vi "serial.Read.vi"(8 "error in":errorcluster, 11 "VISA in":refnum<visa-resource-name>) -> (0 "error out":errorcluster, 2 "msg":string)   [LabVIEW 2020]
uses:
  ecc83fa6-065f-4ed5-ad9c-77edae2b4f3b.vi
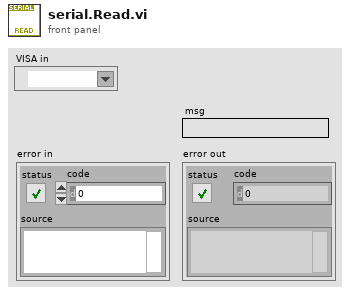
[diagram p1: front panel]
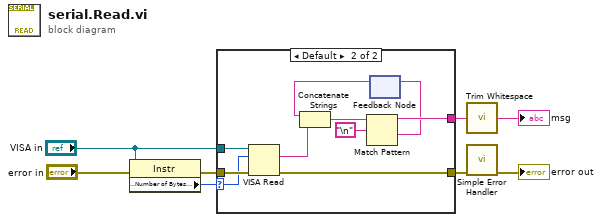
[diagram p0: block diagram]
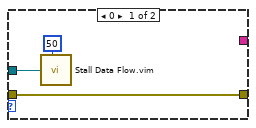
[diagram p2: hidden frame]
diagram:
  n1 = property class="Instr"(reference="VISA in", error in="error in") -> (error out=w6:errorcluster, "Serial Settings:Number of Bytes at Serial Port"=w7:u32)  [unwired: 1 out]
  n2 = case shown="Default" w7 {
    selector: w7 -> [_ w19]
    tunnel: w6 -> [w9 w21]
    tunnel: "VISA in" -> [w11 w20]
    tunnel: [w9 w18] -> w4
    tunnel: [_ w16] -> w3
    frame 0 {
      n3 = call "Stall Data Flow.vim"("value in"=w11, "milliseconds to wait"=u32 50) -> ()  [unwired: 2 out]
    }
    frame Default {
      n4 = VISA Read(VISA resource name=w20, byte count=w19, error in (no error)=w21) -> (read buffer=w13:string, error out=w18:errorcluster)  [unwired: 2 out]
      n5 = feedback #1() -> (w12:string)  [unwired: 1 in]
      n6 = Concatenate Strings(w12, w13) -> (w14:string)
      n7 = Match Pattern(string=w14, regular expression="\n") -> (before substring=w16:string, after substring=w15:string)  [unwired: 1 in, 2 out]
      n8 = feedback-in #1(w15) -> ()
    }
  }
  n9 = call <vilib>:"Trim Whitespace.vi"("string"=w3) -> ("trimmed string"=→"msg":string)  [unwired: 1 in]
  n10 = call <vilib>:"Simple Error Handler.vi"("error in (no error)"=w4) -> ("error out"=→"error out":errorcluster)  [unwired: 4 in, 4 out]
